vi "Render.vi"(8 "error in (no error)":errorcluster, 10 "String in":string, 11 "IRenderable in":refnum<class "IRenderable.lvclass">) -> (0 "error out":errorcluster, 2 "String out":string, 3 "IRenderable out":refnum<class "IRenderable.lvclass">)   [LabVIEW 2021, in "Markdown.lvlib" / "IRenderable.lvclass"]
uses:
  IRenderable.lvclass
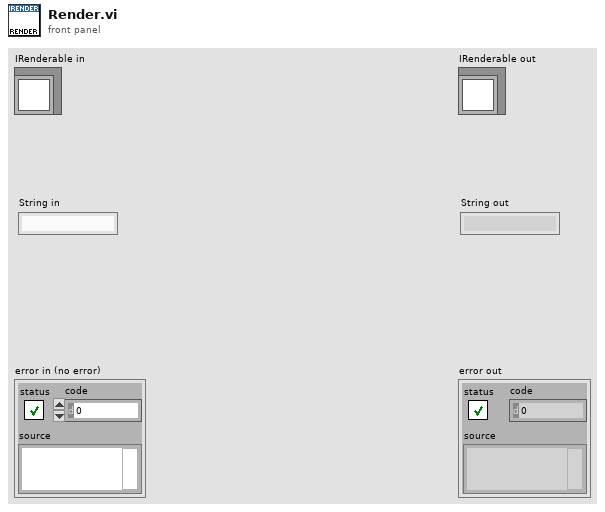
[diagram p1: front panel]
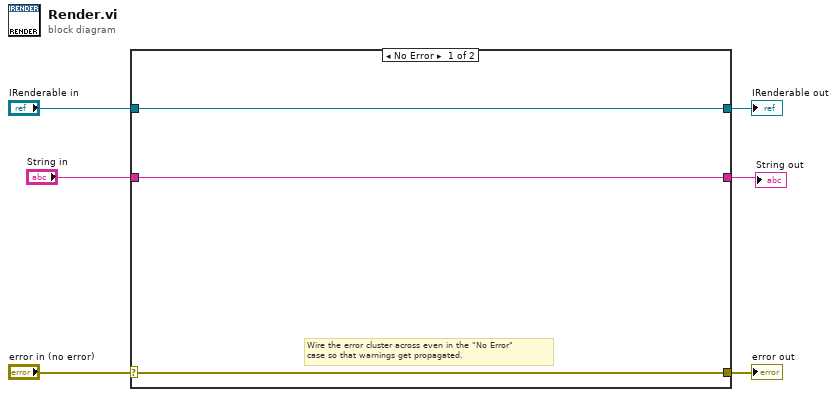
[diagram p0: block diagram]
diagram:
  n1 = case shown="No Error" "error in (no error)" {
    selector: "error in (no error)" -> [w8 w12]
    tunnel: [w8 w12] -> w5
    tunnel: [w9 w11] -> w3
    tunnel: "IRenderable in" -> [w9 w11]
    tunnel: "String in" -> [w7 w10]
    tunnel: [w7 w10] -> w1
    frame No Error {
      # "Wire the error cluster across even in the \"No Error\"\ncase so that warnings get propagated."
    }
    frame Error {
    }
  }
  "error out" <- w5
  "IRenderable out" <- w3
  "String out" <- w1
